vi "Initialize Device.vi"(11 "dir":string) -> (2 "function return":u32, 3 "dir out":string)   [LabVIEW 2018, in "AndorSDK.lvlib"]
doc: "EXPNETTYPE unsigned int WINAPI InitializeDevice(char * dir);"
uses:
  AndorSDK.lvlib
  ATMCD32D.dll
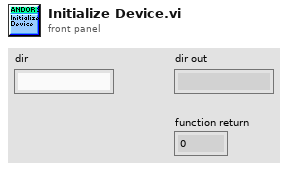
[diagram p1: front panel]
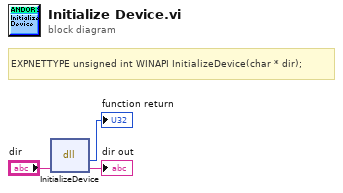
[diagram p0: block diagram]
diagram:
  # "EXPNETTYPE unsigned int WINAPI InitializeDevice(char * dir);"
  n1 = dll-call lib="PTH2babs E\nPersönliches02 - Arbeit03-HiwijobsLabviewCodelibANDOR\tAndor SDK\nATMCD32D.*" fn="InitializeDevice"("dir"="dir") -> (→"function return":u32, "dir"=→"dir out":string)  [unwired: 3 in, 2 out]
